vi "tx.vi"() -> ()   [LabVIEW 2020]
panel:
  in  "String":string
  in  "Serial Init":T1={"Puerto Serial"="", "baud rate (9600)"=9600, "data bits (8)"=8, "parity (0:none)"=enum."None", "error in (no error)"={"status"=FALSE, "code"=0, "source"=""}, "stop bits (10: 1 bit)"=10, "flow control (0:none)"=0} {"flow control (0:none)" items=["None", "XON/XOFF", "RTS/CTS", "XON/XOFF & RTS/CTS", "DTR/DSR", "XON/XOFF & DTR/DSR"]; "stop bits (10: 1 bit)" items=["1.0"=10, "1.5"=15, "2.0"=20]; "data bits (8)" min=5 max=8 step=1}
  in  "stop":bool
  # "Trasnmisor Serial"
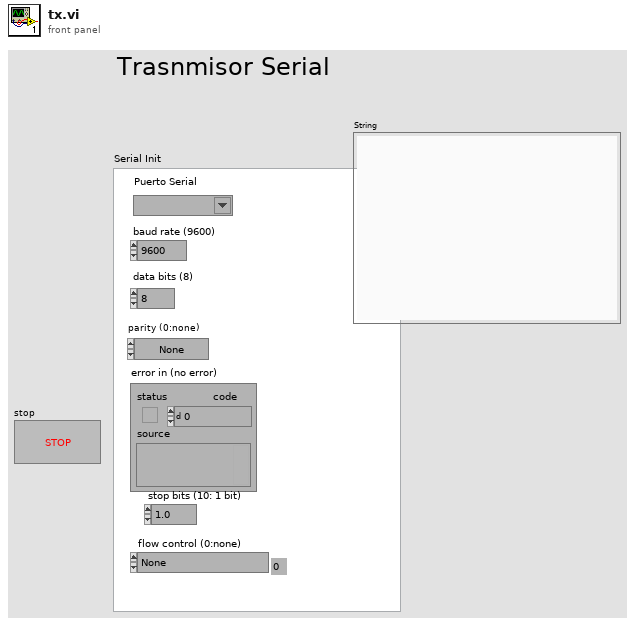
[diagram p1: front panel]
types:
  T1 = cluster{"Puerto Serial":refnum<visa-resource-name>, "baud rate (9600)":u32, "data bits (8)":u16, "parity (0:none)":enum16{"None", "Odd", "Even", "Mark", "Space"}, "error in (no error)":errorcluster, "stop bits (10: 1 bit)":u16, "flow control (0:none)":u16}
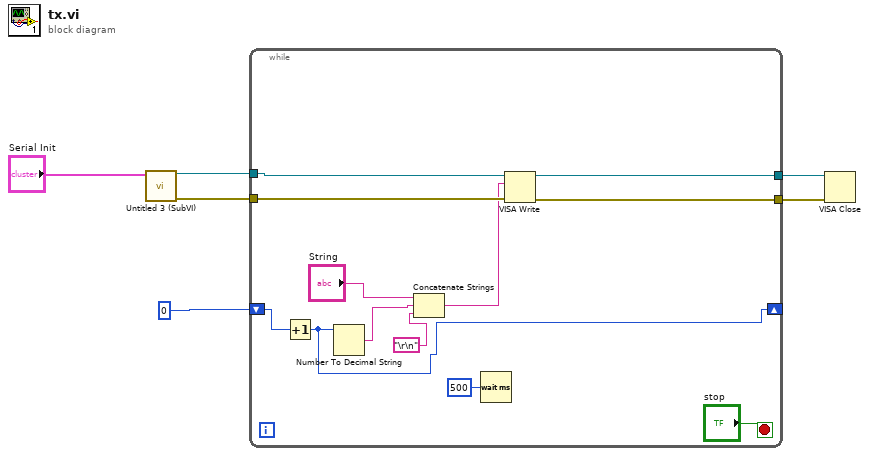
[diagram p0: block diagram]
diagram:
  n1 = call "Untitled 3 (SubVI).vi"("Serial Init"="Serial Init") -> ("error out"=w4:errorcluster, "VISA Refnum out"=w5:refnum<visa-resource-name>)  [unwired: 9 in]
  n2 = while {
    tunnel: w5 -> [w16]
    tunnel: w4 -> [w15]
    tunnel: [w14] -> w2
    tunnel: [w13] -> w3
    shift-right: [w7] -> _
    shift-left: 0 -> [w12]
    stop <- "stop" stop-if-true
    n3 = Increment(x=w12) -> (x+1=w7:i32)
    n4 = Number To Decimal String(number=w7) -> (decimal integer string=w11:string)  [unwired: 1 in]
    n5 = Concatenate Strings("String", w11, "\r\n") -> (w8:string)
    n6 = Wait (ms)(milliseconds to wait=u32 500) -> ()  [unwired: 1 out]
    n7 = VISA Write(VISA resource name=w16, write buffer=w8, error in (no error)=w15) -> (VISA resource name out=w14:refnum<visa-resource-name>, error out=w13:errorcluster)  [unwired: 1 out]
  }
  n8 = VISA Close(VISA resource name=w2, error in (no error)=w3) -> ()  [unwired: 1 out]
